vi "View-Parallel-Port-Data.vi"() -> ()   [LabVIEW 2016]
uses:
  <vilib>/Utility/file.llb/Write Delimited Spreadsheet (I64).vi
panel:
  out "data string":string
  out "size(s)":i32[](array[numeric])
  out "min value":u16
  out "max value":u16
  out "appended array 3":u16[][](array[numeric]) format="%x"
  out "appended array 2":dbl[][](array[numeric])
  out "Input":dbl[](array[numeric])
  in  "Chanal":u16
  out "Numeric 2":i32
  in  "y":dbl
  in  "Chanal Gain":dbl[](array[numeric])=[1.0, 1.0, 1.0, 1.0]
  in  "Signal Freq [kHz]":dbl[](array[numeric])=[1561.0, 1561.0, 1561.0, 1561.0]
  out "sum":i32
  out "appended array":i32[](array[numeric])
  out "Numeric":i32
  out "error out":errorcluster
  out "Waveform Graph":waveform(dbl)[](graph)
  in  "File":path
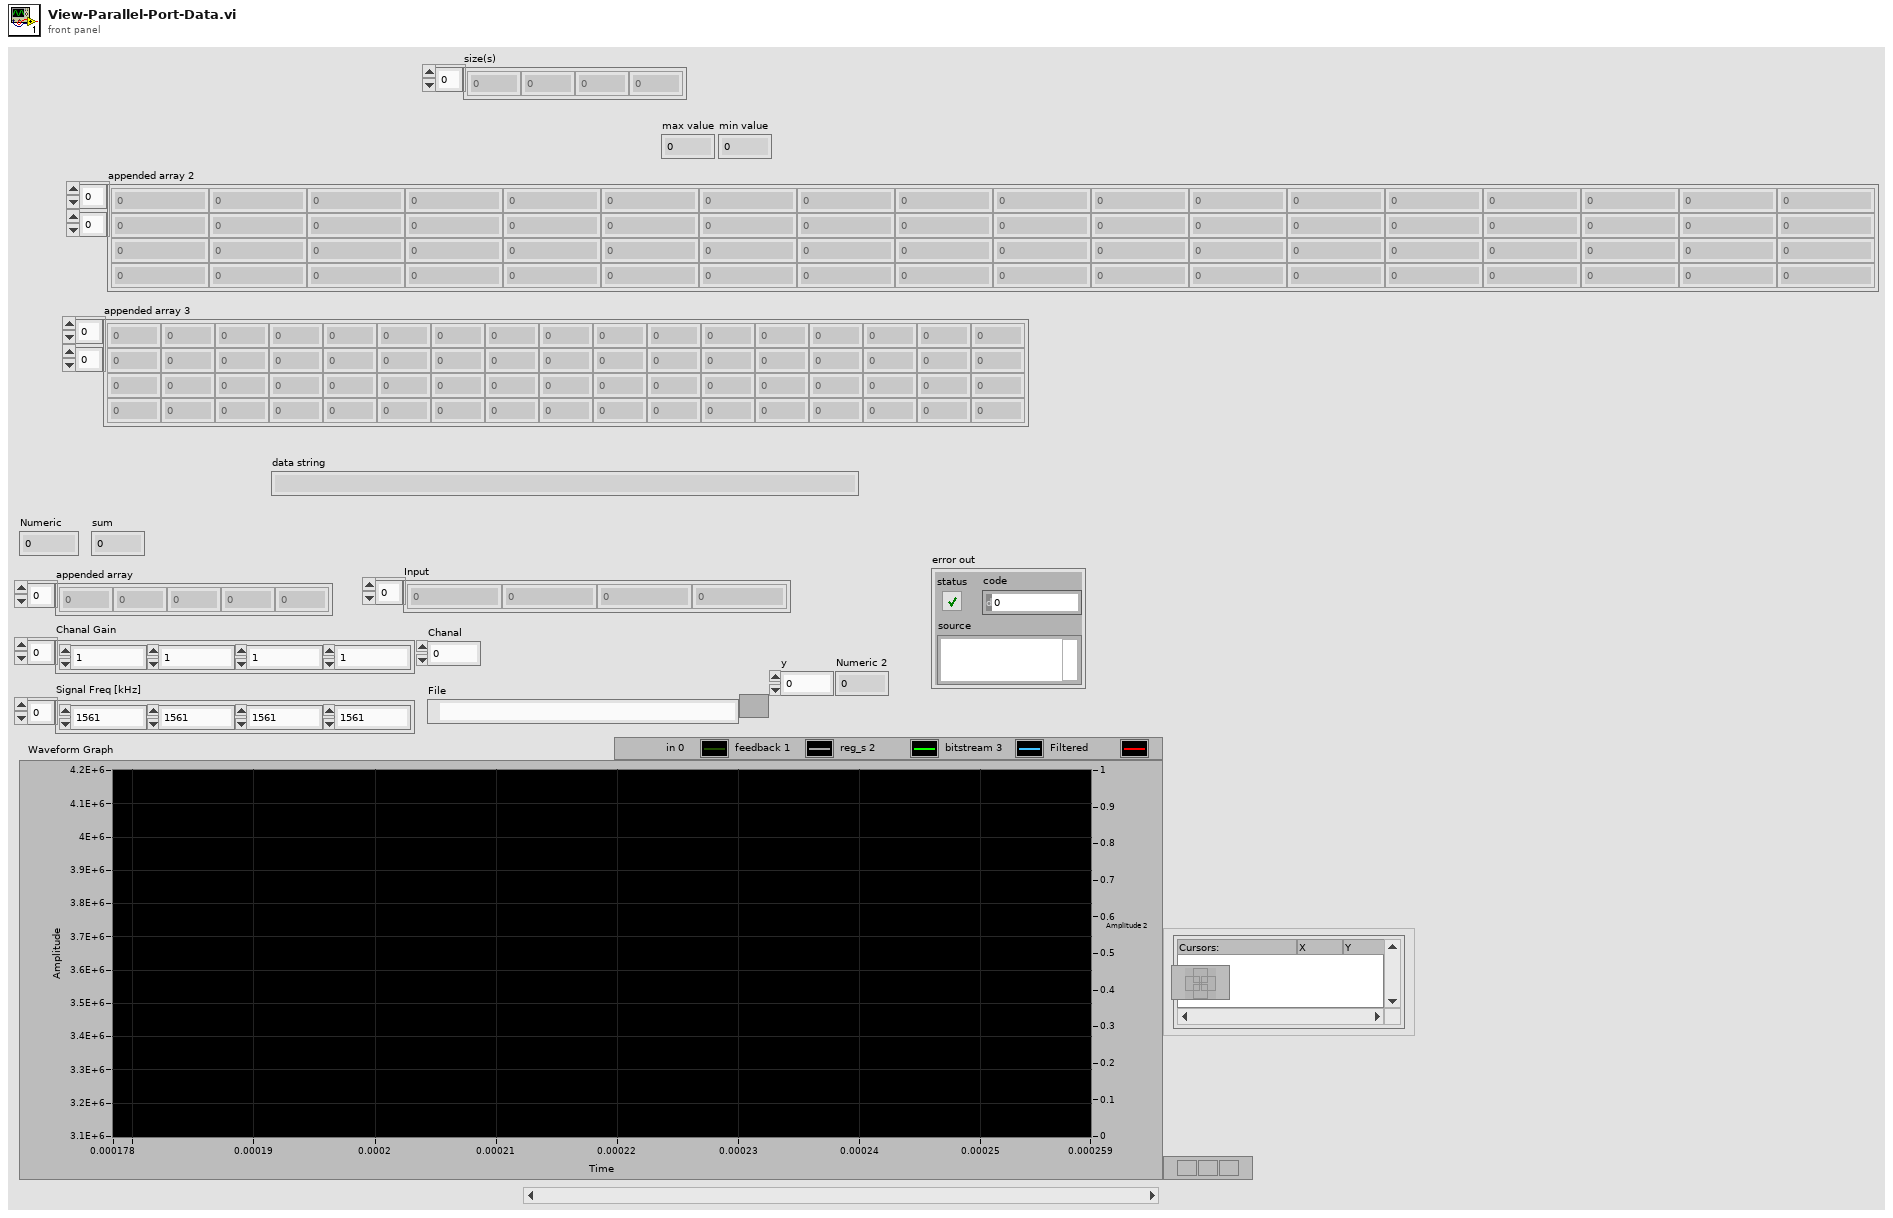
[diagram p1: front panel]
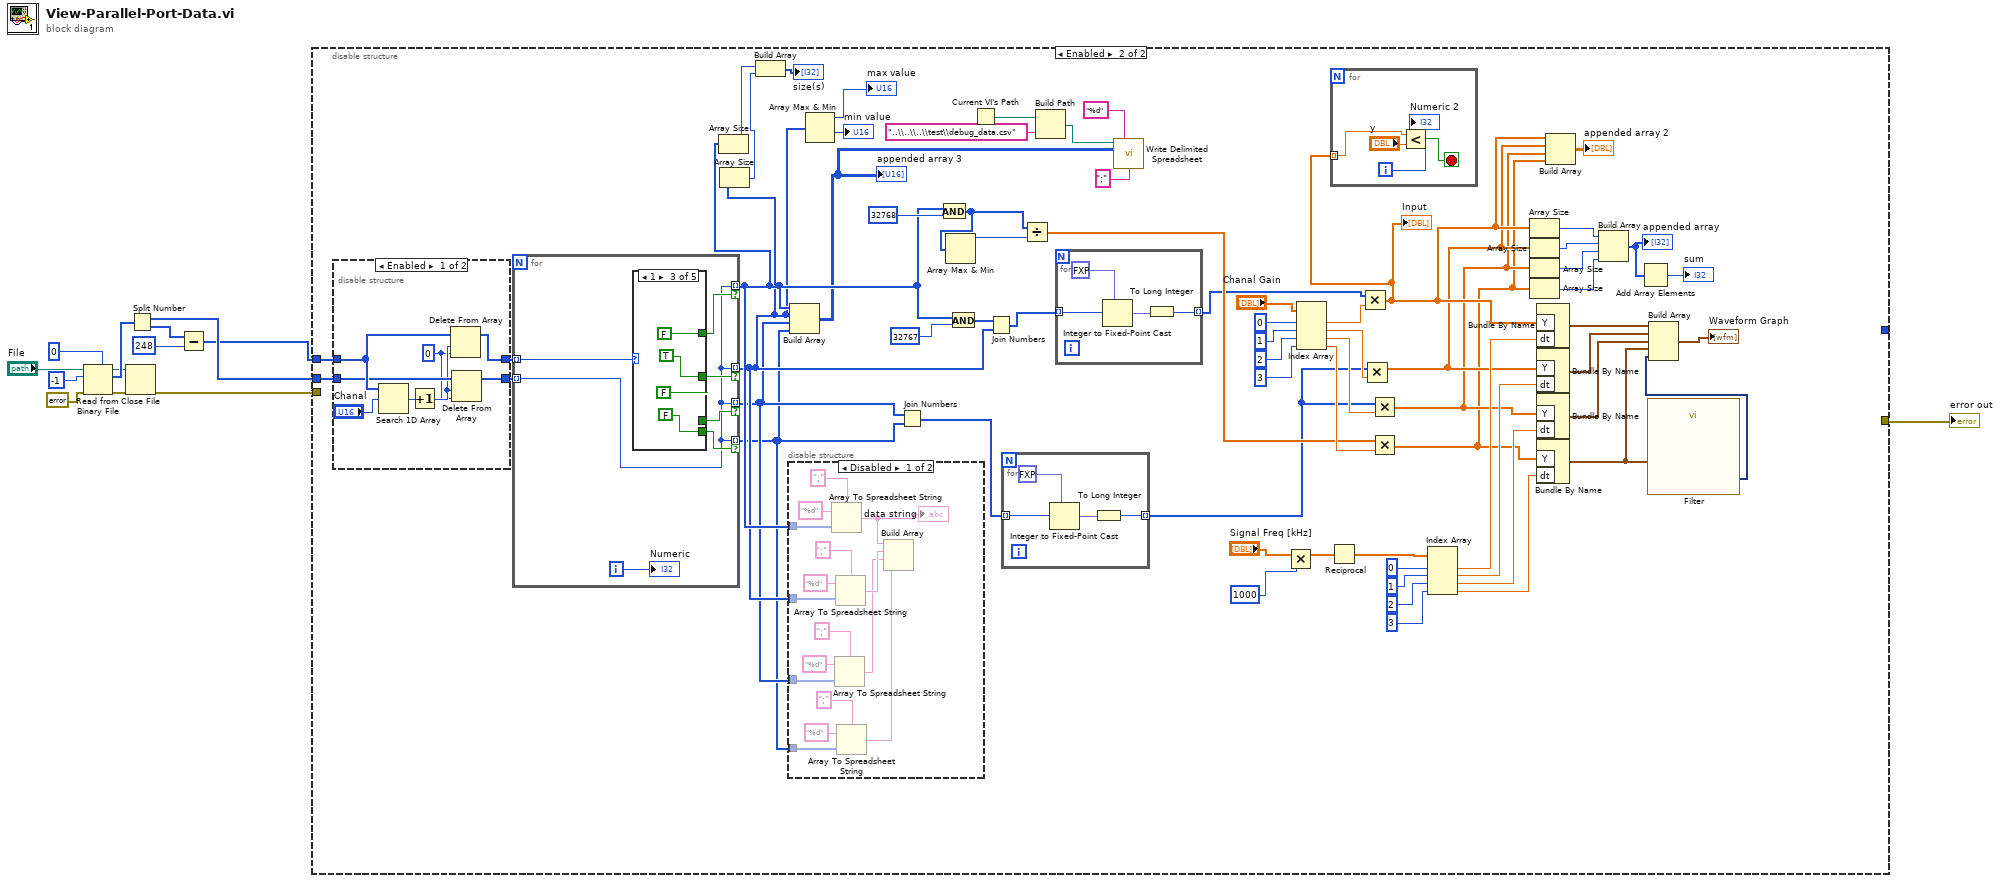
[diagram p0: block diagram]
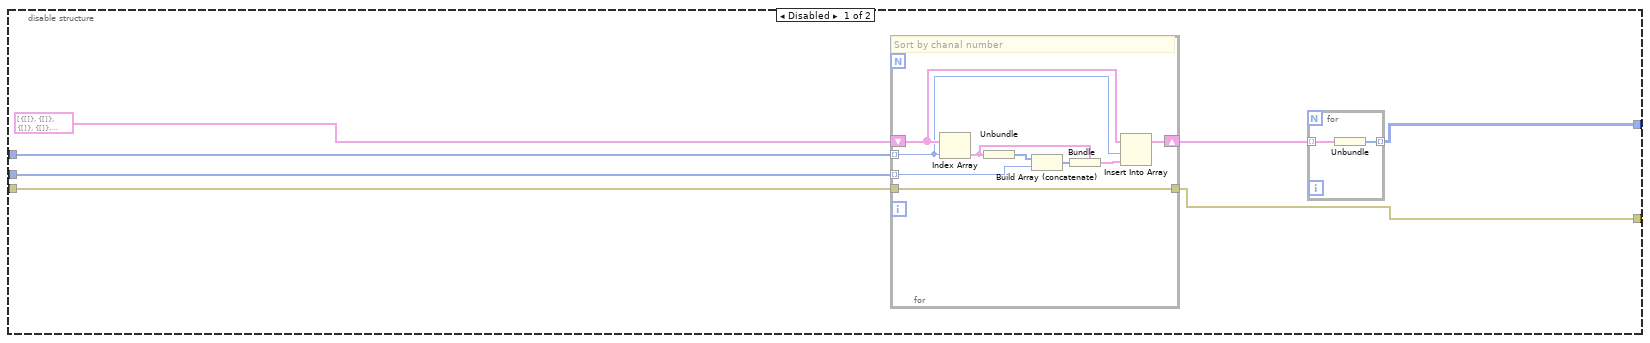
[diagram p2: hidden frame]
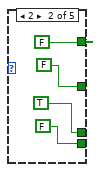
[diagram p6: hidden frame]
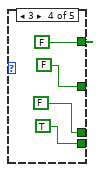
[diagram p7: hidden frame]
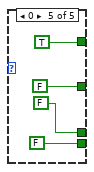
[diagram p8: hidden frame]
diagram:
  n1 = Read from Binary File(5:u32 0, 8:errorcluster {"status"=FALSE, "code"=0, "source"=""} ("error in"), 10:-1 ("count (1)"), 11:"File") -> (0:w5:errorcluster, 2:w13:u32[], 3:w6:refnum<file>)  [unwired: 2 in, 1 out]
  n2 = Close File(refnum=w6, error in=w5) -> (error out=w12:errorcluster)  [unwired: 1 out]
  n3 = Split Number(x=w13) -> (hi(x)=w8:u16[], lo(x)=w11:u16[])
  n4 = Subtract(x=w11, y=u16 248) -> (x-y=w7:u16[])
  n5 = disable-structure shown="Enabled" {
    disable-tunnel: w12 -> [w20 _]
    disable-tunnel: w7 -> [w19 w65]
    disable-tunnel: [w16 _] -> _
    disable-tunnel: [w15 _] -> w10
    disable-tunnel: w8 -> [w14 w63]
    frame Disabled {
      n6 = for {
        tunnel: w20 -> [w24]
        tunnel: w14 -> [w22] mode=indexing
        shift-right: [w25] -> w17
        shift-left: cluster{u16[]}[] [{[]}, {[]}, {[]}, {[]}, {[0]}] -> [w29]
        tunnel: w19 -> [w28] mode=indexing
        tunnel: [w24] -> w15
        # "Sort by chanal number"
        n7 = Index Array(array=w29, index=w28) -> (element=w27:cluster{u16[]})
        n8 = Unbundle(w27) -> (w23:u16[])
        n9 = Build Array (concatenate)(w23, w22) -> (w21:u16[])
        n10 = Bundle(cluster=w27, w21) -> (w26:cluster{u16[]})
        n11 = Insert Into Array(array=w29, index=w28, new element=w26) -> (w25:cluster{u16[]}[])
      }
      n12 = for {
        tunnel: w17 -> [w31] mode=indexing
        tunnel: [w30] -> w16 mode=indexing
        n13 = Unbundle(w31) -> (w30:u16[])
      }
    }
    frame Enabled {
      n14 = disable-structure shown="Enabled" {
        disable-tunnel: w65 -> [w129 w132]
        disable-tunnel: [w127 w132] -> w64
        disable-tunnel: w63 -> [w126 w131]
        disable-tunnel: [w125 w131] -> w62
        frame Enabled {
          w123 = 0 ("index")
          n15 = Search 1D Array(1D array=w129, element="Chanal") -> (index of element=w128:i32)  [unwired: 1 in]
          n16 = Increment(x=w128) -> (x+1=w124:i32)
          n17 = Delete From Array(array=w129, length=w124, index=w123) -> (array with subset deleted=w127:u16[])  [unwired: 1 out]
          n18 = Delete From Array(array=w126, length=w124, index=w123) -> (array with subset deleted=w125:u16[])  [unwired: 1 out]
        }
        frame Disabled {
        }
      }
      n19 = for {
        tunnel: w64 -> [w139] mode=indexing
        tunnel: w62 -> [w133] mode=indexing
        tunnel: [w133] -> w41 mode=indexing if=w134
        tunnel: [w133] -> w40 mode=indexing if=w138
        tunnel: [w133] -> w39 mode=indexing if=w137
        tunnel: [w133] -> w38 mode=indexing if=w136
        i -> [w135]
        n20 = case shown="1" w139 {
          tunnel: [_ FALSE FALSE FALSE TRUE] -> w134
          tunnel: [_ FALSE TRUE FALSE FALSE] -> w138
          tunnel: [_ TRUE FALSE FALSE FALSE] -> w137
          tunnel: [_ FALSE FALSE TRUE FALSE] -> w136
          frame 4, Default {
          }
          frame 2 {
          }
          frame 1 {
          }
          frame 3 {
          }
          frame 0 {
          }
        }
        "Numeric" <- w135
      }
      n21 = Array Size(array=w41) -> (size(s)=w44:i32)
      n22 = Array Size(array=w40) -> (size(s)=w43:i32)
      n23 = Build Array(w44, w43) -> (→"size(s)":i32[])
      n24 = disable-structure shown="Disabled" {
        disable-tunnel: w41 -> [w112 _]
        disable-tunnel: w40 -> [w107 _]
        disable-tunnel: w39 -> [w102 _]
        disable-tunnel: w38 -> [w101 _]
        frame Disabled {
          n25 = Array To Spreadsheet String(delimiter (Tab)=";", array=w112, 3:"%d" ("format string")) -> (spreadsheet string=w109:string)
          "data string" <- w109
          n26 = Array To Spreadsheet String(delimiter (Tab)=";", array=w102, 3:"%d" ("format string")) -> (spreadsheet string=w100:string)
          n27 = Array To Spreadsheet String(delimiter (Tab)=";", array=w107, 3:"%d" ("format string")) -> (spreadsheet string=w108:string)
          n28 = Array To Spreadsheet String(delimiter (Tab)=";", array=w101, 3:"%d" ("format string")) -> (spreadsheet string=w99:string)
          n29 = Build Array(w109, w108, w100, w99) -> ()  [unwired: 1 out]
        }
        frame Enabled {
        }
      }
      n30 = Build Array(w41, w40, w39, w38) -> (w37:u16[][])
      "appended array 3" <- w37
      n31 = Array Max & Min(array=w40) -> (max value=→"max value":u16, min value=→"min value":u16)  [unwired: 2 out]
      n32 = Join Numbers(hi=w39, lo=w38) -> ((hi.lo)=w53:u32[])
      n33 = And(x=w41, y=32768) -> (x .and. y?=w57:i32[])
      n34 = Array Max & Min(array=w57) -> (max value=w56:i32)  [unwired: 3 out]
      n35 = And(x=w41, y=u16 32767) -> (x .and. y?=w60:u16[])
      n36 = Current VI's Path() -> (path=w34:path)
      n37 = Join Numbers(hi=w60, lo=w40) -> ((hi.lo)=w55:u32[])
      n38 = for {
        tunnel: w53 -> [w118] mode=indexing
        tunnel: [w116] -> w52 mode=indexing
        n39 = Integer to Fixed-Point Cast(fixed-point type=fxp<+/-,31,31> 0.0, integer=w118) -> (fixed-point=w117:fxp<+/-,31,31>)
        n40 = To Long Integer(number=w117) -> (32bit integer=w116:i32)
      }
      n41 = Divide(x=w57, y=w56) -> (x/y=w58:dbl[])
      n42 = Build Path(base path=w34, name or relative path="..\\..\\..\\test\\debug_data.csv") -> (appended path=w32:path)
      n43 = for {
        tunnel: w55 -> [w122] mode=indexing
        tunnel: [w120] -> w54 mode=indexing
        n44 = Integer to Fixed-Point Cast(fixed-point type=fxp<+/-,31,31> 0.0, integer=w122) -> (fixed-point=w121:fxp<+/-,31,31>)
        n45 = To Long Integer(number=w121) -> (32bit integer=w120:i32)
      }
      n46 = call-poly <vilib>:"Write Delimited Spreadsheet.vi"("file path (dialog if empty)"=w32, "format (%d)"="%d" ("format string"), "2D data"=w37, "delimiter (\\t)"=";" ("delimiter (\\t)")) -> ()  [unwired: 10 in, 2 out]
      n47 = Multiply(x="Signal Freq [kHz]", y=1000 ("dt")) -> (x*y=w79:dbl[])
      n48 = Index Array(array="Chanal Gain", index #1=0 ("index"), index #2=1 ("index"), index #3=2 ("index"), index #4=3 ("index")) -> (element #1=w70:dbl, element #2=w68:dbl, element #3=w67:dbl, element #4=w66:dbl)
      n49 = Reciprocal(x=w79) -> (1/x=w80:dbl[])
      n50 = Multiply(x=w54, y=w70) -> (x*y=w51:dbl[])
      "Input" <- w51
      n51 = for {
        tunnel: w51 -> [w159] mode=indexing
        i -> [w156]
        stop <- w157 stop-if-true
        n52 = Less?(x=w159, y="y") -> (x < y?=w157:bool)
        "Numeric 2" <- w156
      }
      n53 = Multiply(x=w52, y=w68) -> (x*y=w50:dbl[])
      n54 = Multiply(x=w52, y=w67) -> (x*y=w49:dbl[])
      n55 = Multiply(x=w58, y=w66) -> (x*y=w48:dbl[])
      n56 = Index Array(array=w80, index #1=0 ("index"), index #2=1 ("index"), index #3=2 ("index"), index #4=3 ("index")) -> (element #1=w92:dbl, element #2=w91:dbl, element #3=w90:dbl, element #4=w89:dbl)
      n57 = Array Size(array=w51) -> (size(s)=w98:i32)
      n58 = Array Size(array=w50) -> (size(s)=w97:i32)
      n59 = Array Size(array=w49) -> (size(s)=w96:i32)
      n60 = Array Size(array=w48) -> (size(s)=w95:i32)
      n61 = Bundle By Name("Y"=w51, "dt"=w92) -> (w84:waveform(dbl))  [unwired: 1 in]
      n62 = Bundle By Name("Y"=w50, "dt"=w91) -> (w83:waveform(dbl))  [unwired: 1 in]
      n63 = Bundle By Name("Y"=w49, "dt"=w90) -> (w77:waveform(dbl))  [unwired: 1 in]
      n64 = Bundle By Name("Y"=w48, "dt"=w89) -> (w75:waveform(dbl))  [unwired: 1 in]
      n65 = Build Array(w51, w50, w49, w48) -> (→"appended array 2":dbl[][])
      n66 = Build Array(w98, w97, w96, w95) -> (w94:i32[])
      "appended array" <- w94
      n67 = Add Array Elements(numeric array=w94) -> (sum=→"sum":i32)
      n68 = call "Filter"("Signal"=w75) -> ("Filtered Signal"=w76:dynamicdata)  [unwired: 9 in, 1 out]
      n69 = Build Array(w84, w83, w77, w75, w76) -> (→"Waveform Graph":waveform(dbl)[])
    }
  }
  "error out" <- w10
